vi "ConcatenateMessages.vi"(2 "Messages 2":u8[](array[numeric]), 3 "Messages":u8[](array[numeric])) -> (0 "Combined Messages":u8[](array[numeric]))   [LabVIEW 2012]
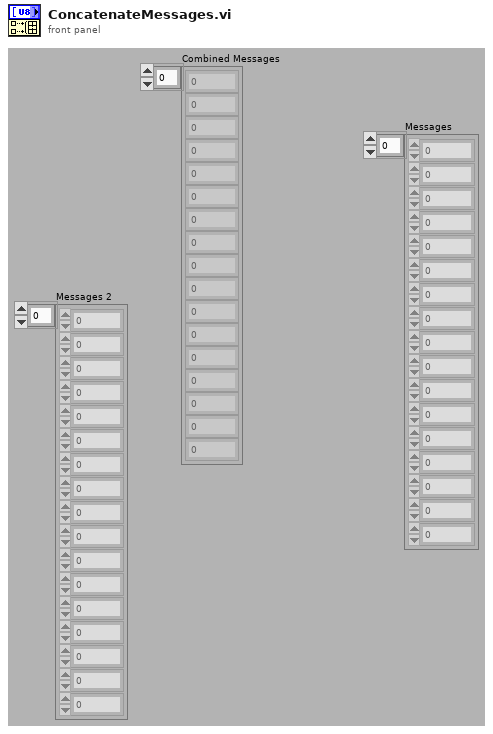
[diagram p1: front panel]
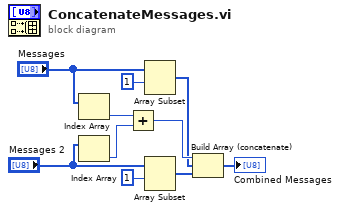
[diagram p0: block diagram]
diagram:
  n1 = Index Array(array="Messages") -> (element=w1:u8)  [unwired: 1 in]
  n2 = Index Array(array="Messages 2") -> (element=w9:u8)  [unwired: 1 in]
  n3 = Add(x=w1, y=w9) -> (x+y=w8:u8)
  n4 = Array Subset(array="Messages", index=1) -> (w7:u8[])  [unwired: 1 in]
  n5 = Array Subset(array="Messages 2", index=1) -> (w4:u8[])  [unwired: 1 in]
  n6 = Build Array (concatenate)(w8, w7, w4) -> (→"Combined Messages":u8[])
